vi "Table-Resize table.vi"(8 "error in (no error)":errorcluster, 9 "Number of columns":i32, 10 "Number of rows":i32, 11 "Table ref in":refnum<vi>) -> (0 "error out":errorcluster, 2 "Resized table":string[][](array[string]), 3 "Table ref out":refnum<vi>)   [LabVIEW 2013]
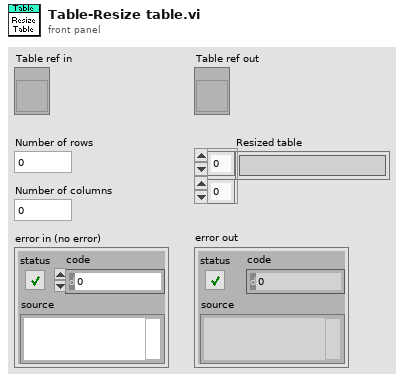
[diagram p1: front panel]
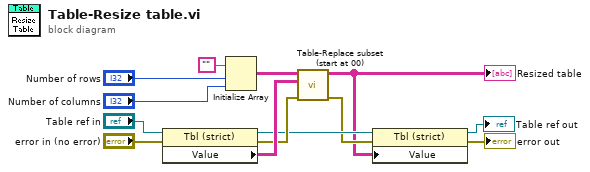
[diagram p0: block diagram]
diagram:
  n1 = property on="Property Node" class="Tbl (strict)"(reference="Table ref in", error in="error in (no error)") -> (reference out=w5:refnum<vi>, error out=w7:errorcluster, "Value"=w8:string[][])
  n2 = Initialize Array("", "Number of rows", "Number of columns") -> (w12:string[][])
  n3 = call "Table-Replace subset (start at 00).vi"("error in (no error)"=w7, "Table to replace with"=w8, "Original table"=w12) -> ("error out"=w4:errorcluster, "Table out"=w2:string[][])  [unwired: 7 in]
  "Resized table" <- w2
  n4 = property on="Property Node" class="Tbl (strict)"(reference=w5, error in=w4, "Value"=w2) -> (reference out=→"Table ref out":refnum<vi>, error out=→"error out":errorcluster)
